vi "Schedule Clay Robot.vi"(6 "max geodes in":u8=24, 7 "max time in":u8=24, 8 "costs in":T1, 9 "data value reference":refnum<data-value>, 10 "stack in":refnum<queue>, 11 "mine in":refnum<class "Mine.lvclass">) -> (0 "costs out":T1, 1 "data value reference":refnum<data-value>, 2 "stack out":refnum<queue>, 3 "mine out":refnum<class "Mine.lvclass">, 4 "max geodes out":u8, 5 "max time out":u8)   [LabVIEW 2021, in "d19.lvlib" / "Mine.lvclass"]
uses:
  Mine.lvclass
  Mine.lvclass/Mine.ctl
  <vilib>/Utility/miscctls.llb/LVMapReplaceAction.ctl
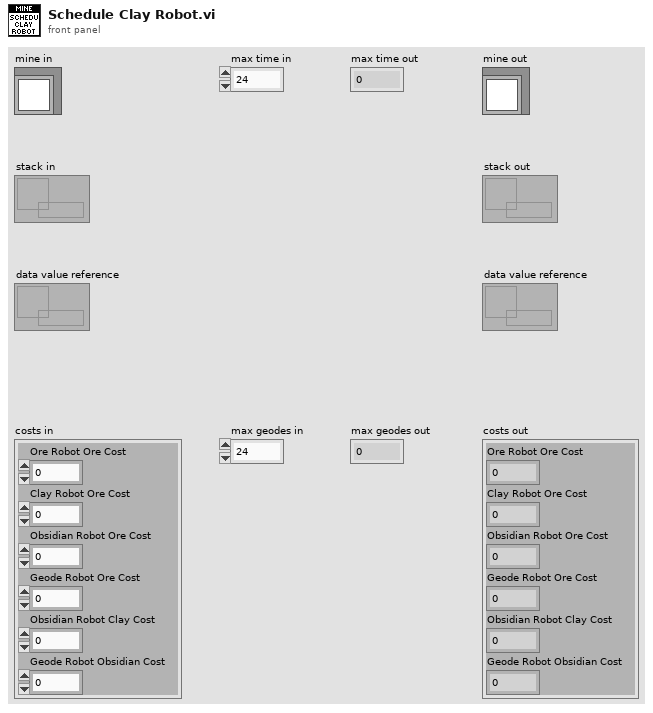
[diagram p1: front panel]
types:
  T1 = cluster{"Ore Robot Ore Cost":u8, "Clay Robot Ore Cost":u8, "Obsidian Robot Ore Cost":u8, "Geode Robot Ore Cost":u8, "Obsidian Robot Clay Cost":u8, "Geode Robot Obsidian Cost":u8}
  T2 = typedef "LVMapReplaceAction.ctl" = enum32{"Modify Entry only if found", "Add or Modify Entry", "Delete Entry"}
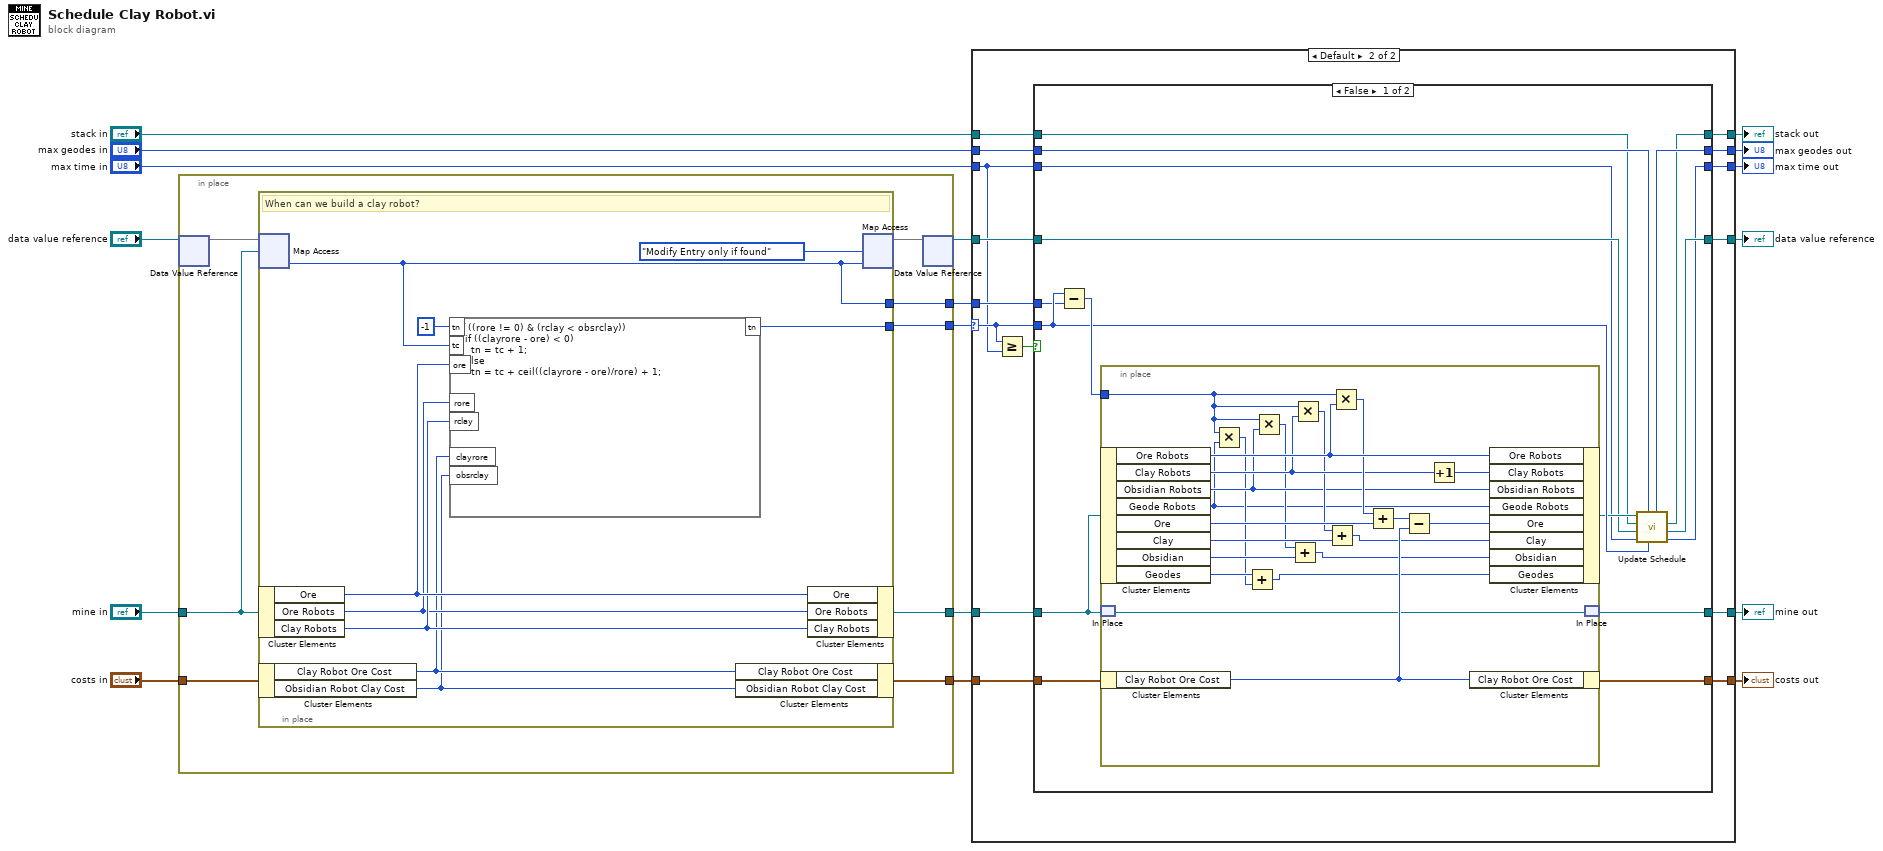
[diagram p0: block diagram]
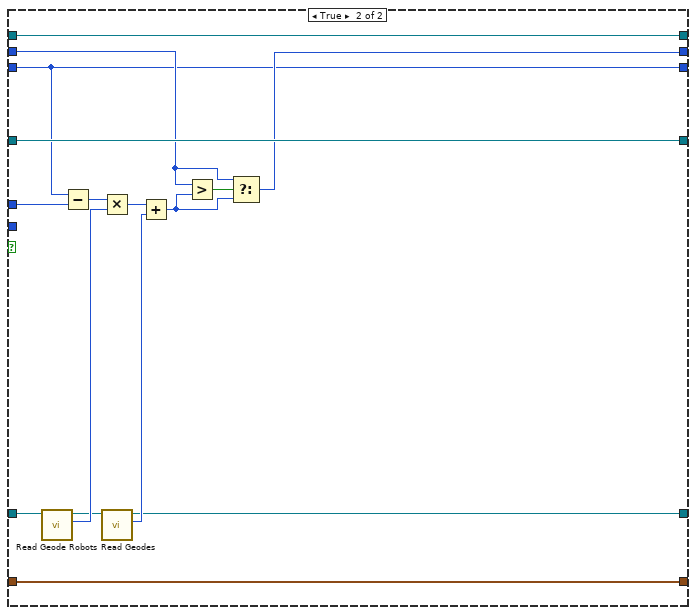
[diagram p3: hidden frame]
diagram:
  n1 = in-place {
    in-place-border: "costs in" -> [w25]
    in-place-border: "mine in" -> [w24]
    in-place-border: [w23] -> w15
    in-place-border: [w22] -> w11
    in-place-border: [w21] -> w10
    in-place-border: [w20] -> w6
    n2 = in-place-dvr #1("data value reference") -> (w19:map{refnum<class "Mine.lvclass">, u8})  [unwired: 1 out]
    n3 = in-place {
      in-place-border: [w27] -> w23
      in-place-border: [w26] -> w20
      # "When can we build a clay robot?"
      n4 = in-place-map #2(w19, w24) -> (w26:u8)  [unwired: 1 in, 1 out]
      n5 = in-place-cluster #3(w24) -> ("Ore"=w33:u8, "Ore Robots"=w31:u8, "Clay Robots"=w32:u8)
      n6 = in-place-cluster #4(w25) -> ("Clay Robot Ore Cost"=w30:u8, "Obsidian Robot Clay Cost"=w29:u8)
      n7 = formula code="if ((rore != 0) & (rclay < obsrclay))\n  if ((clayrore - ore) < 0)\n    tn = tc + 1;\n  else \n    tn = tc + ceil((clayrore - ore)/rore) + 1;"("tc"=w26, "clayrore"=w30, "obsrclay"=w29, "ore"=w33, "rore"=w31, "rclay"=w32, "tn"=i8 -1) -> ("tn"=w27:i8)
      n8 = in-place-cluster #4("Clay Robot Ore Cost"=w30, "Obsidian Robot Clay Cost"=w29) -> (w22:T1)
      n9 = in-place-cluster #3("Ore"=w33, "Ore Robots"=w31, "Clay Robots"=w32) -> (w21:refnum<class "Mine.lvclass">)
      n10 = in-place-map #2(w26, LVMapReplaceAction."Modify Entry only if found" ("action")) -> (w18:map{refnum<class "Mine.lvclass">, u8})  [unwired: 2 out]
    }
    n11 = in-place-dvr #1(w18) -> (w1:refnum<data-value>)  [unwired: 1 out]
  }
  n12 = case shown="Default" w15 {
    selector: w15 -> [_ w43]
    tunnel: "stack in" -> [w40 w55]
    tunnel: [w40 w54] -> w13
    tunnel: [w37 w53] -> w12
    tunnel: w11 -> [w35 w52]
    tunnel: w10 -> [w36 w51]
    tunnel: [w35 w50] -> w9
    tunnel: [w36 w49] -> w8
    tunnel: "max time in" -> [w38 w42]
    tunnel: w6 -> [_ w48]
    tunnel: "max geodes in" -> [w39 w47]
    tunnel: [w39 w46] -> w4
    tunnel: [w38 w45] -> w3
    tunnel: w1 -> [w37 w44]
    frame -1 {
    }
    frame Default {
      n13 = Greater Or Equal?(x=w43, y=w42) -> (x >= y?=w41:bool)
      n14 = case shown="False" w41 {
        tunnel: w44 -> [w58 w108]
        tunnel: [w61 w108] -> w53
        tunnel: w55 -> [w59 w107]
        tunnel: [w60 w107] -> w54
        tunnel: w52 -> [w71 w106]
        tunnel: w51 -> [w68 w96]
        tunnel: [w70 w106] -> w50
        tunnel: [w67 w94] -> w49
        tunnel: w42 -> [w57 w101]
        tunnel: w48 -> [w63 w100]
        tunnel: w47 -> [w66 w103]
        tunnel: [w65 w104] -> w46
        tunnel: [w56 w101] -> w45
        tunnel: w43 -> [w64 _]
        frame False {
          n15 = Subtract(x=w64, y=w63) -> (x-y=w69:u8)
          n16 = in-place {
            in-place-border: w69 -> [w72]
            n17 = in-place-cluster #5(w68) -> ("Ore Robots"=w86:u8, "Clay Robots"=w82:u8, "Obsidian Robots"=w80:u8, "Geode Robots"=w75:u8, "Ore"=w92:u8, "Clay"=w89:u8, "Obsidian"=w79:u8, "Geodes"=w88:u8)
            n18 = in-place-match #6(w68) -> (w87:refnum<class "Mine.lvclass">)
            n19 = in-place-cluster #7(w71) -> ("Clay Robot Ore Cost"=w91:u8)
            n20 = Multiply(x=w72, y=w75) -> (x*y=w76:u8)
            n21 = Add(x=w88, y=w76) -> (x+y=w74:u8)
            n22 = Multiply(x=w72, y=w80) -> (x*y=w77:u8)
            n23 = Add(x=w77, y=w79) -> (x+y=w78:u8)
            n24 = Multiply(x=w72, y=w82) -> (x*y=w81:u8)
            n25 = Add(x=w81, y=w89) -> (x+y=w84:u8)
            n26 = Multiply(x=w72, y=w86) -> (x*y=w83:u8)
            n27 = Add(x=w83, y=w92) -> (x+y=w85:u8)
            n28 = Subtract(x=w85, y=w91) -> (x-y=w90:u8)
            n29 = Increment(x=w82) -> (x+1=w73:u8)
            n30 = in-place-cluster #7("Clay Robot Ore Cost"=w91) -> (w70:T1)
            n31 = in-place-cluster #5("Ore Robots"=w86, "Clay Robots"=w73, "Obsidian Robots"=w80, "Geode Robots"=w75, "Ore"=w90, "Clay"=w84, "Obsidian"=w78, "Geodes"=w74) -> (w62:refnum<class "Mine.lvclass">)
            n32 = in-place-match #6(w87) -> (w67:refnum<class "Mine.lvclass">)
          }
          n33 = call "Update Schedule.vi"("new time"=w64, "max geodes in"=w66, "max time in"=w57, "map in"=w58, "stack in"=w59, "Mine in"=w62) -> ("max time out"=w56:u8, "map out"=w61:refnum<data-value>, "stack out"=w60:refnum<queue>, "max geodes out"=w65:u8)  [unwired: 1 in, 1 out]
        }
        frame True {
          n34 = call "Read Geode Robots.vi"("Mine in"=w96) -> ("Geode Robots"=w98:u8, "Mine out"=w95:refnum<class "Mine.lvclass">)  [unwired: 9 in]
          n35 = Subtract(x=w101, y=w100) -> (x-y=w99:u8)
          n36 = Multiply(x=w99, y=w98) -> (x*y=w97:u8)
          n37 = call "Read Geodes.vi"("Mine in"=w95) -> ("Geodes"=w102:u8, "Mine out"=w94:refnum<class "Mine.lvclass">)  [unwired: 9 in]
          n38 = Add(x=w97, y=w102) -> (x+y=w93:u8)
          n39 = Greater?(x=w103, y=w93) -> (0:w105:bool)
          n40 = Select(t=w103, s=w105, f=w93) -> (s? t:f=w104:u8)
        }
      }
    }
  }
  "stack out" <- w13
  "data value reference" <- w12
  "costs out" <- w9
  "mine out" <- w8
  "max geodes out" <- w4
  "max time out" <- w3
